vi "Remap Demo both + ROIs.vi"() -> ()   [LabVIEW 2018]
uses:
  <vilib>/vision/NI_Vision_Development_Module.lvlib
  RemapDemo/LV_RemapOpenCV/x64/Release/LVRemapOpenCV.dll
panel:
  in  "Angle (degrees)":dbl=2.0 format="%.2f"
  out "Grid Dst":T1(plugin-control)
  out "Image Dst":T1(plugin-control)
  out "Pattern":T1(plugin-control)
  out "Image src":T1(plugin-control)
  out "Grid":T1(plugin-control)
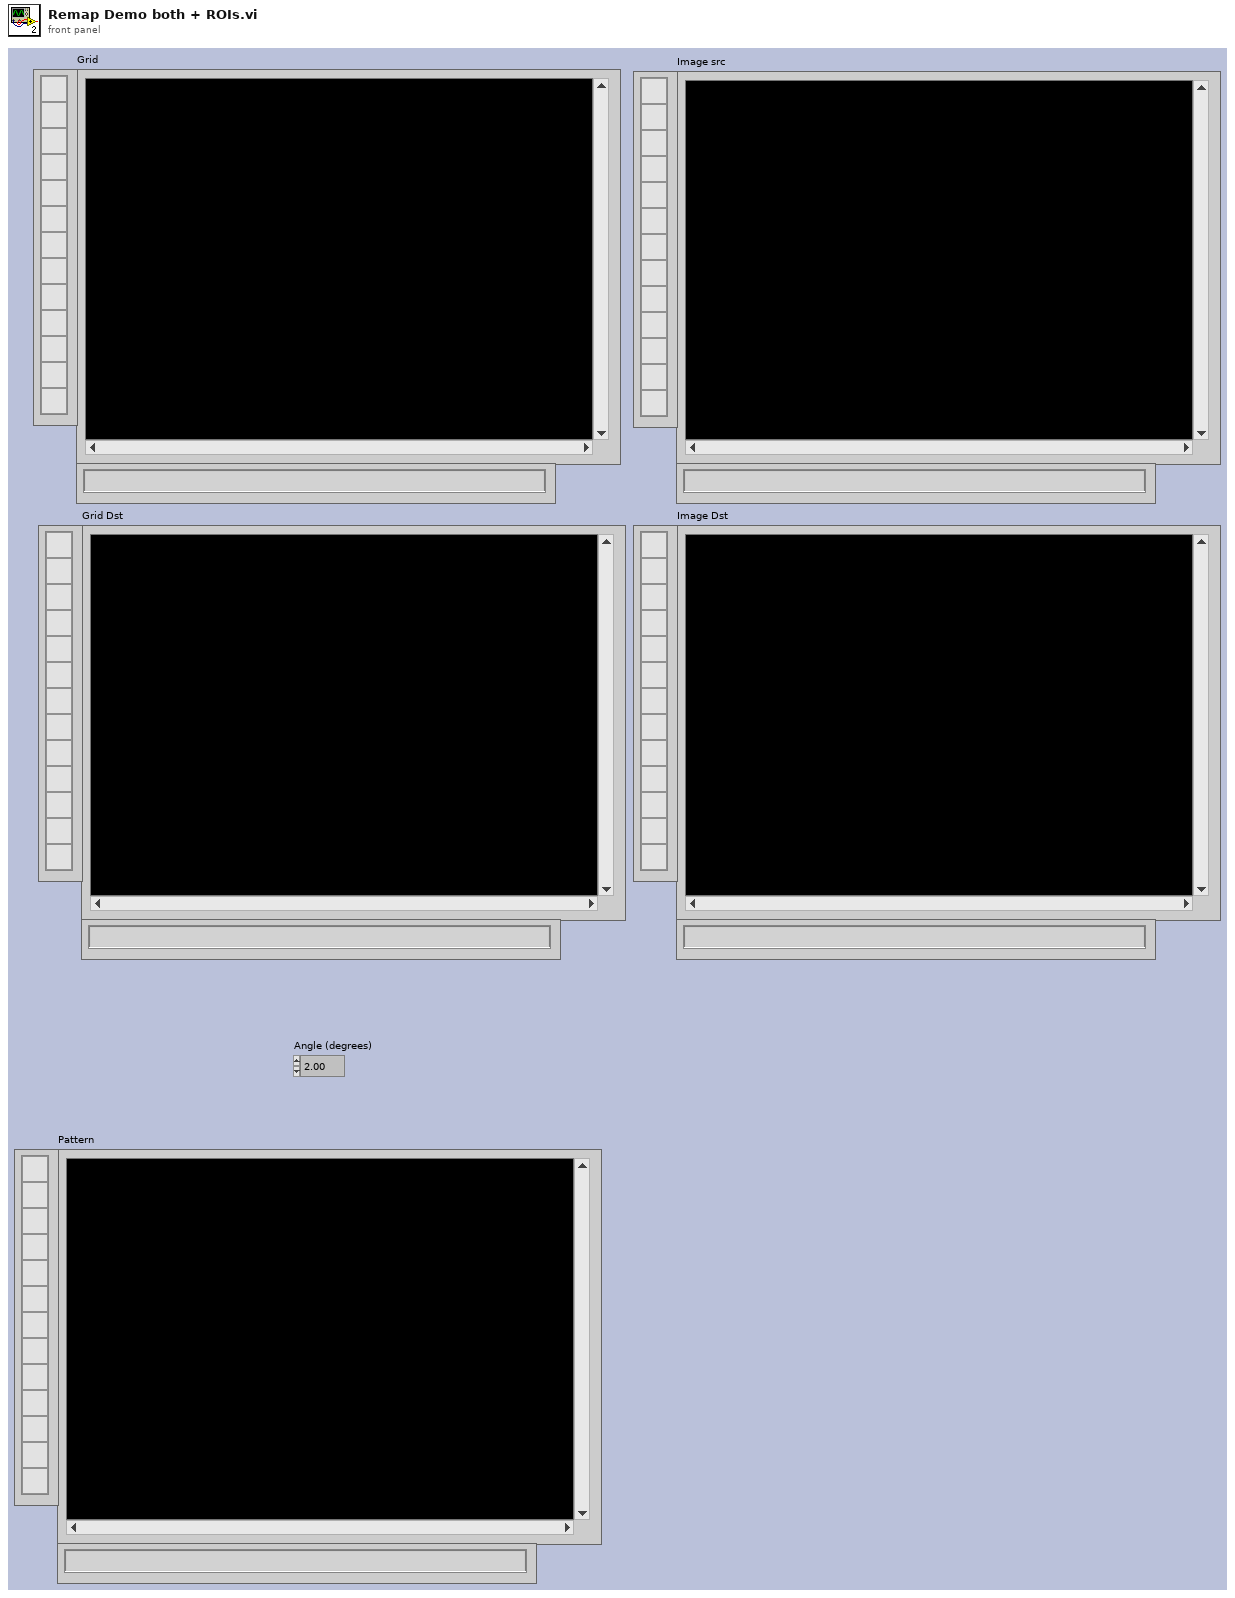
[diagram p1: front panel]
types:
  T1 = typedef "IMAQ Image.ctl" = refnum<image>
  T2 = typedef "Image Unit" = enum32{"Undefined", "Angström", "Micrometer", "Millimeter", "Centimeter", "Meter", "Kilometer", "Microinch", "Inch", "Feet", "Nautical miles", "Standard miles", "Steps"}
  T3 = typedef "Particle Parameters" = i32
  T4 = cluster{"Measurement Parameter":T3, "Range Lower Value":dbl, "Range Upper Value":dbl, "Range":bool, "Measurement Type":bool}[]
  T5 = typedef "Calibration Reference Points.ctl" = cluster{"Pixel Coordinates":cluster{"X":dbl, "Y":dbl}[], "Real World Coordinates":cluster{"X":dbl, "Y":dbl}[], "Unit":T2, "Image Size":cluster{"X":u32, "Y":u32}}
  T6 = cluster{"Global Rectangle":i32[], "Contours":cluster{"Contour Type":u32, "ROI Type":u32, "Points":i32[]}[]}
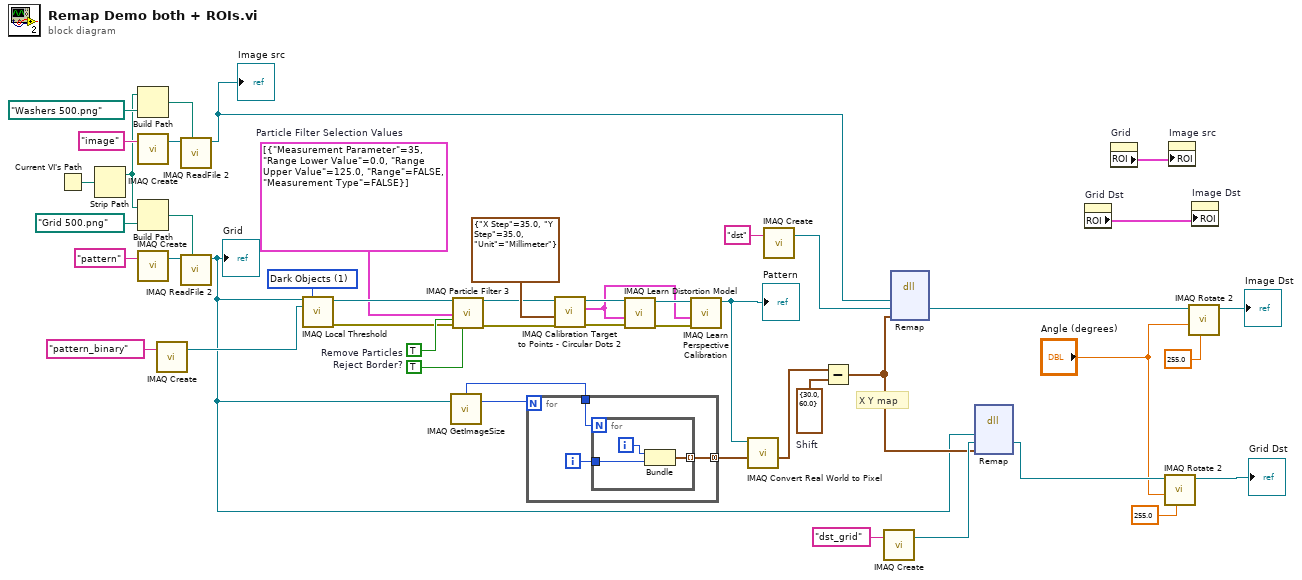
[diagram p0: block diagram]
diagram:
  w20 = cluster{"X":sgl, "Y":sgl} {"X"=30.0, "Y"=60.0}  # Shift
  w30 = T4 [{"Measurement Parameter"=35, "Range Lower Value"=0.0, "Range Upper Value"=125.0, "Range"=FALSE, "Measurement Type"=FALSE}]  # Particle Filter Selection Values
  w33 = TRUE  # Remove Particles
  w32 = TRUE  # Reject Border?
  w38 = u32 1 items=["Bright Objects", "Dark Objects"] ("Look For (Bright Objects)")
  # "X Y map"
  n1 = Current VI's Path() -> (path=w48:path)
  n2 = Strip Path(path=w48) -> (stripped path=w39:path)  [unwired: 1 out]
  n3 = Build Path(base path=w39, name or relative path=path "Washers 500.png") -> (appended path=w42:path)
  n4 = call "IMAQ Create"("Image Name"="image") -> ("New Image"=w43:T1)  [unwired: 4 in, 1 out]
  n5 = Build Path(base path=w39, name or relative path=path "Grid 500.png") -> (appended path=w45:path)
  n6 = call "IMAQ Create"("Image Name"="pattern") -> ("New Image"=w44:T1)  [unwired: 4 in, 1 out]
  n7 = call "IMAQ Create"("Image Name"="pattern_binary") -> ("New Image"=w11:T1)  [unwired: 4 in, 1 out]
  n8 = call "IMAQ ReadFile 2"("File Path"=w42, "Image"=w43) -> ("Image Out"=w19:T1)  [unwired: 5 in, 4 out]
  "Image src" <- w19
  n9 = call "IMAQ ReadFile 2"("File Path"=w45, "Image"=w44) -> ("Image Out"=w10:T1)  [unwired: 5 in, 4 out]
  "Grid" <- w10
  n10 = call "IMAQ Local Threshold"("Image Src"=w10, "Look For (Bright Objects)"=w38, "Image Dst"=w11) -> ("Image Dst Out"=w31:T1, "error out"=w29:errorcluster)  [unwired: 6 in, 5 out]
  n11 = call "IMAQ GetImageSize"("Image"=w10) -> ("Y Resolution"=w17:i32, "X Resolution"=w18:i32)  [unwired: 3 in, 1 out]
  n12 = call "IMAQ Particle Filter 3"("Image Src"=w31, "Selection Values"=w30, "Keep/Remove Particles (F)"=w33, "error in (no error)"=w29, "Reject Border? (F)"=w32) -> ("Image Dst Out"=w25:T1, "error out"=w28:errorcluster)  [unwired: 4 in, 5 out]
  n13 = for {
    N: w17 -> [_]
    tunnel: [w50] -> w22 mode=concatenating
    tunnel: w18 -> [w49]
    i -> [w51]
    n14 = for {
      N: w49 -> [_]
      tunnel: w51 -> [w53]
      tunnel: [w52] -> w50 mode=indexing
      i -> [w54]
      n15 = Bundle(w54, w53) -> (w52:cluster{i32, i32})  [unwired: 1 in]
    }
  }
  n16 = call "IMAQ Calibration Target to Points - Circular Dots 2"("error in (no error)"=w28, "Grid Descriptor"=cluster{"X Step":sgl, "Y Step":sgl, "Unit":T2} {"X Step"=35.0, "Y Step"=35.0, "Unit"=enum."Millimeter"}, "Target Image"=w25) -> ("error out"=w27:errorcluster, "Reference Points"=w35:T5, "Target Image (dup)"=w37:T1)  [unwired: 6 in]
  n17 = call "IMAQ Learn Distortion Model"("error in (no error)"=w27, "Reference Points"=w35, "Calibration Template Image"=w37) -> ("error out"=w26:errorcluster, "Calibration Template Image Out"=w36:T1)  [unwired: 3 in, 4 out]
  n18 = call "IMAQ Learn Perspective Calibration"("error in (no error)"=w26, "Reference Points"=w35, "Calibration Template Image"=w36) -> ("Calibration Template Image Out"=w16:T1)  [unwired: 1 in, 7 out]
  "Pattern" <- w16
  n19 = call "IMAQ Convert Real World to Pixel"("Array of Real World Coordinates"=w22, "Calibrated Image"=w16) -> ("Array of Pixel Coordinates"=w21:cluster{"X":sgl, "Y":sgl}[])  [unwired: 4 in, 5 out]
  n20 = call "IMAQ Create"("Image Name"="dst") -> ("New Image"=w23:T1)  [unwired: 4 in, 1 out]
  n21 = Subtract(x=w21, y=w20) -> (x-y=w13:cluster{"X":sgl, "Y":sgl}[])
  n22 = call "IMAQ Create"("Image Name"="dst_grid") -> ("New Image"=w14:T1)  [unwired: 4 in, 1 out]
  n23 = dll-call lib="C:/Users/108003658/OneDrive - Baker Hughes/Desktop/RemapDemo/LV_RemapOpenCV/x64/Release/LVRemapOpenCV.dll" fn="Remap"("arg1"=w19, "arg2"=w23, "XYmap"=w13) -> ("arg2"=w7:T1)  [unwired: 6 in, 2 out]
  n24 = dll-call lib="C:/Users/108003658/OneDrive - Baker Hughes/Desktop/RemapDemo/LV_RemapOpenCV/x64/Release/LVRemapOpenCV.dll" fn="Remap"("arg1"=w10, "Image dst 2"=w14, "XYmap"=w13) -> ("Image dst 2"=w9:T1)  [unwired: 6 in, 2 out]
  n25 = property on="Grid Dst" class="ImageControl"() -> ("ROI"=w1:T6)  [unwired: 2 in, 2 out]
  n26 = property on="Grid" class="ImageControl"() -> ("ROI"=w2:T6)  [unwired: 2 in, 2 out]
  n27 = call "IMAQ Rotate 2"("Replace Value"=sgl 255.0, "Angle (degrees)"="Angle (degrees)", "Image Src"=w9) -> ("Image Dst Out"=→"Grid Dst":T1)  [unwired: 7 in, 1 out]
  n28 = property on="Image src" class="ImageControl"("ROI"=w2) -> ()  [unwired: 2 in, 2 out]
  n29 = call "IMAQ Rotate 2"("Replace Value"=sgl 255.0, "Angle (degrees)"="Angle (degrees)", "Image Src"=w7) -> ("Image Dst Out"=→"Image Dst":T1)  [unwired: 7 in, 1 out]
  n30 = property on="Image Dst" class="ImageControl"("ROI"=w1) -> ()  [unwired: 2 in, 2 out]
